vi "Analog Input - N Channels - 1 Sample.vi"() -> ()   [LabVIEW 2019]
uses:
  <vilib>/myRIO/Common/Instrument Driver Framework/ELVIS III v1.0/AI/vis/ELVIS III v1.0 Close AI.vi
  <vilib>/myRIO/Common/Instrument Driver Framework/myRIO v1.0/UART/vis/myRIO v1.0 Close UART.vi
  <vilib>/myRIO/Common/Instrument Driver Framework/ELVIS III v1.0/AI/vis/ELVIS III v1.0 Unreserve AI.vi
  <vilib>/myRIO/Common/Instrument Driver Framework/ELVIS III v1.0/AI/vis/ELVIS III v1.0 Build MUX Configuration AI.vi
  <vilib>/Utility/error.llb/Error Cluster From Error Code.vi
  <vilib>/myRIO/Common/Instrument Driver Framework/ELVIS III v1.0/AI/vis/ELVIS III v1.0 Read AI.vi
  <vilib>/myRIO/Common/Instrument Driver Framework/ELVIS III v1.0/Resource Manager/vis/ELVIS III v1.0 Unreserve Channel List.vi
  <vilib>/myRIO/Common/Instrument Driver Framework/myRIO v1.0/myRIO v1.0 Close.vi
  <vilib>/myRIO/Common/Instrument Driver Framework/Utilities/vis/FPGA Ref Manager.vi
  <vilib>/myRIO/Common/Instrument Driver Framework/ELVIS III v1.0/ELVIS III v1.0 Reset FPGA.vi
  <vilib>/myRIO/Common/Instrument Driver Framework/myRIO v1.0/IRQ/vis/myRIO v1.0 IRQ Info FGV.vi
  <vilib>/myRIO/Common/Instrument Driver Framework/myRIO v1.0/IRQ/vis/myRIO v1.0 Timer IRQ Info FGV.vi
  <vilib>/myRIO/Common/Instrument Driver Framework/myRIO v1.0/IRQ/vis/myRIO v1.0 ISR Agent.vi
  <vilib>/myRIO/Instrument Drivers/Utilities/vis/Reset Index.vi
  <vilib>/myRIO/Common/Instrument Driver Framework/myRIO v1.0/Resource Manager/vis/myRIO v1.0 Block Write Resource Manager.vi
  <vilib>/myRIO/Instrument Drivers/Utilities/Utilities.lvlib
  <vilib>/myRIO/Instrument Drivers/Onboard IO/AI/AI.lvlib
panel:
  out "Analog Data":cluster{"A/AI0":dbl, "A/AI1":dbl}(graph)
  in  "Stop":bool
  # "ELVIS III Control IO"
  # "模拟输入N通道"
  # "Overview: Acquires single point voltage values per loop iteration from Bank A, Channels 0 and 1 (A/AI0 and A/AI1).\nInstructions:\n1. Connect A/AI0 and A/AI1 to valid signals.\n2. Run the VI."
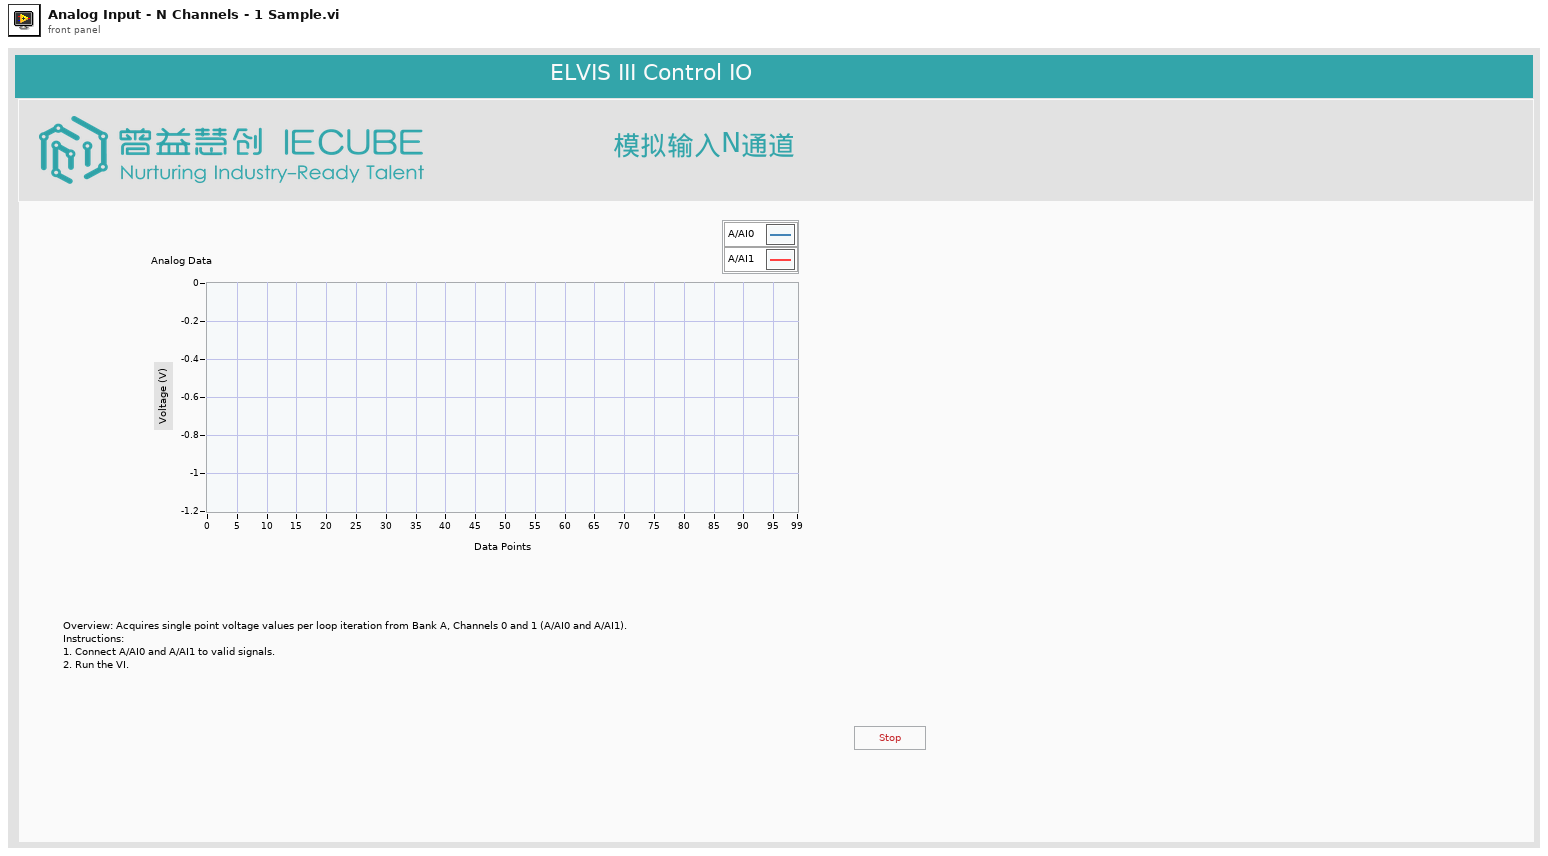
[diagram p1: front panel]
types:
  T1 = typedef "AI.lvlib/AI Reference.ctl" = cluster{"myRIO Reference":T2, "AI Channels List":T6, "AI Scaling Constants List":T8}
  T2 = typedef "myRIO Generic Hardware Reference.ctl" = cluster{"myRIO Model":T3, "myRIO Hardware Reference":T4}
  T3 = typedef "Hardware Version Enum.ctl" = enum16{"Unknown", "myRIO-1900", "myRIO-1950", "roboRIO", "NI ELVIS RIO CM", "ELVIS III"}
  T4 = typedef "myRIO v1.0 Reference.ctl" = cluster{"Generic FPGA Reference":T5, "Allow multiple opens":bool}
  T5 = typedef "Generic FPGA Reference.ctl" = refnum<k20>
  T6 = typedef "AI Channels List.ctl" = T7[]
  T7 = typedef "AI Channels Enum.ctl" = enum16{"Not Connected", "AudioIn/Left", "AudioIn/Right", "C/AI0", "C/AI1", "A/AI0", "A/AI1", "A/AI2", "A/AI3", "A/AI4", "A/AI5", "A/AI6", "A/AI7", "B/AI0", "B/AI1", "B/AI2", "B/AI3", "B/AI4", "B/AI5", "B/AI6", "B/AI7", "AI/AI0", "AI/AI1", "AI/AI2", "AI/AI3", "A/AI0 (DIFF)", "A/AI1 (DIFF)", "A/AI2 (DIFF)", "A/AI3 (DIFF)", "B/AI0 (DIFF)", "B/AI1 (DIFF)", "B/AI2 (DIFF)", "B/AI3 (DIFF)"}
  T8 = typedef "Analog Scaling Constants List.ctl" = T9[]
  T9 = typedef "Analog Scaling Constants.ctl" = cluster{"LSB Weight (Volts)":dbl, "Offset (Volts)":dbl, "Signed?":bool}
  T10 = cluster{"dbl Scaled Value":dbl, "dbl Scaled Value":dbl}
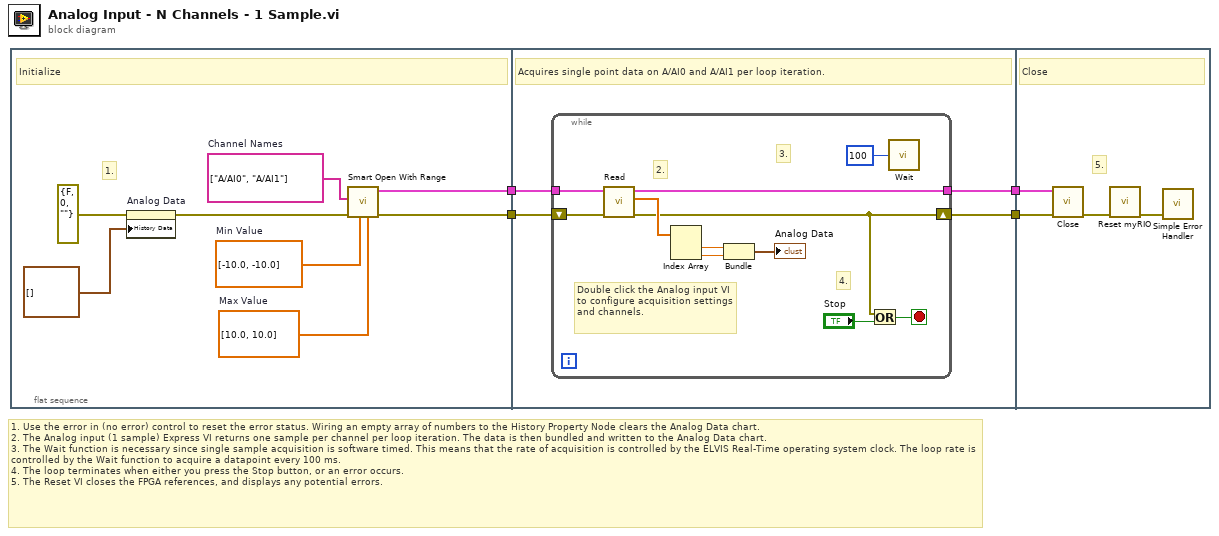
[diagram p0: block diagram]
diagram:
  # "1. Use the error in (no error) control to reset the error status. Wiring an empty array of numbers to the History Property Node clears the Analog Data chart. \n2. The Analog input (1 sample) Express VI returns one sample per channel per loop iteration. The data is then bundled and written to the Analog Data chart.\n3. The Wait function is necessary since single sample acquisition is software timed. This means that the rate of acquisition is controlled by the ELVIS Real-Time operating system clock. The loop rate is controlled by the Wait function to acquire a datapoint every 100 ms.\n4. The loop terminates when either you press the Stop button, or an error occurs.\n5. The Reset VI closes the FPGA references, and displays any potential errors."
  n1 = flat-sequence {
    tunnel: [w6] -> w4
    tunnel: [w5] -> w2
    tunnel: w4 -> [w16]
    tunnel: [w15] -> w3
    tunnel: w2 -> [w14]
    tunnel: [w13] -> w1
    tunnel: w3 -> [w30]
    tunnel: w1 -> [w28]
    frame #0 {
      w10 = dbl[] [10.0, 10.0]  # Max Value
      w9 = dbl[] [-10.0, -10.0]  # Min Value
      w8 = tag[] ["A/AI0", "A/AI1"]  # Channel Names
      # "1."
      # "Initialize"
      n2 = property on="Analog Data" class="WFChart (严格)"(error in=errorcluster {"status"=FALSE, "code"=0, "source"=""} ("error in (no error)"), "History Data"=cluster{"A/AI0":dbl, "A/AI1":dbl}[] []) -> (error out=w7:errorcluster)  [unwired: 1 in, 1 out]
      n3 = call <vilib>:"Smart Open With Range.vi"("Max Value"=w10, "Min Value"=w9, "error in (no error)"=w7, "Channel Names"=w8) -> ("error out"=w6:errorcluster, "AI Ref Out"=w5:T1)  [unwired: 6 in]
    }
    frame #1 {
      # "Acquires single point data on A/AI0 and A/AI1 per loop iteration."
      n4 = while {
        shift-right: [w20] -> w15
        shift-left: w16 -> [w22]
        tunnel: w14 -> [w21]
        tunnel: [w17] -> w13
        stop <- w27 stop-if-true
        # "4."
        # "3."
        # "2."
        # "Double click the Analog input VI to configure acquisition settings and channels."
        n5 = call <vilib>:"Read.vi"("error in (no error)"=w22, "AI Ref In"=w21) -> ("error out"=w20:errorcluster, "Values"=w23:dbl[], "AI Ref Out"=w17:T1)  [unwired: 7 in]
        n6 = Index Array(array=w23) -> (element #1=w19:dbl, element #2=w18:dbl)  [unwired: 2 in]
        n7 = Bundle("dbl Scaled Value"=w19, "dbl Scaled Value"=w18) -> (→"Analog Data":T10)  [unwired: 1 in]
        n8 = Or(x=w20, y="Stop") -> (x .or. y?=w27:bool)
        n9 = call "Wait"("Count(mSec)"=u32 100) -> ()  [unwired: 1 out]
      }
    }
    frame #2 {
      # "5."
      # "Close"
      n10 = call <vilib>:"Close.vi"("error in (no error)"=w30, "AI Ref In"=w28) -> ("error out"=w29:errorcluster)  [unwired: 9 in]
      n11 = call <vilib>:"Reset myRIO.vi"("error in (no error)"=w29) -> ("error out"=w31:errorcluster)  [unwired: 10 in]
      n12 = call <vilib>:"Simple Error Handler.vi"("error in (no error)"=w31) -> ()  [unwired: 4 in, 5 out]
    }
  }
